vi "Setup SMU Channels.vi"(0 "TSM context":T1) -> (15 "error out":errorcluster)   [LabVIEW 2019]
uses:
  <vilib>/NI_TestStand_SemiconductorModule/NI_TestStand_Semiconductor_Module.lvlibp/PinMap/General/SemiconductorModuleContext.ctl
  <instrlib>/niDCPower/nidcpower.llb/niDCPower Sense.ctl
  <instrlib>/niDCPower/nidcpower.llb/niDCPower Aperture Time Units.ctl
  <vilib>/Utility/High Resolution Polling Wait.vi
  Instrument Control/DCPower/SSC DCPower/Source/SSC DCPower Configure Output Connected.vi
  Instrument Control/DCPower/SSC DCPower/Source/SSC DCPower Configure Output Enabled.vi
  <vilib>/NI_TestStand_SemiconductorModule/NI_TestStand_Semiconductor_Module.lvlibp
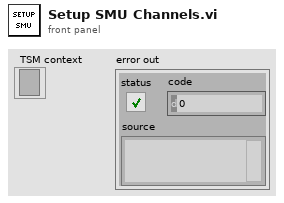
[diagram p1: front panel]
types:
  T1 = typedef "NI_TestStand_Semiconductor_Module.lvlibp/SemiconductorModuleContext.ctl" = refnum<k7>
  T2 = typedef "niDCPower Aperture Time Units.ctl" = i32
  T3 = typedef "niDCPower Sense.ctl" = i32
  T4 = typedef "TSM SSC DCPower.ctl" = cluster{"Pin Query Context":refnum<class "MultiplePinMultipleSessionQueryContext.lvclass">, "SSC":T5[], "Site Numbers":i32[], "Pins":T6[], "Pins Expanded":T8[]}
  T5 = typedef "SSC DCPower.ctl" = cluster{"Session":refnum<k15>, "Chan":string, "Channel List":string}
  T6 = typedef "TSM Pin Information.ctl" = cluster{"Pin":tag, "Type":T7, "Count":i32}
  T7 = typedef "TSM Pin Type Identifier.ctl" = enum8{"DUT Pin", "System Pin", "Pin Group", "Not Determined"}
  T8 = typedef "TSM Expanded Pin Information.ctl" = cluster{"Pin":tag, "Type":T7, "Index":i32}
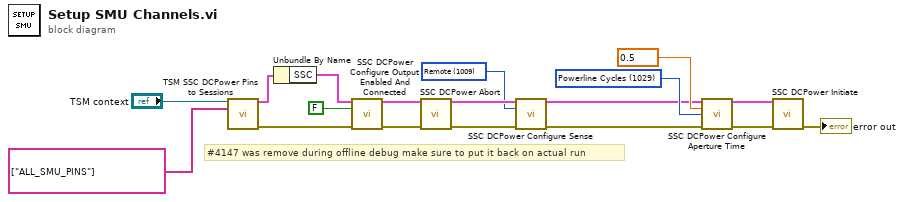
[diagram p0: block diagram]
diagram:
  w4 = T2 1029 items=["Seconds"=1028, "Powerline Cycles"=1029] ("Aperture Time Units")
  w8 = T3 1009 items=["Local"=1008, "Remote"=1009] ("Sense")
  # "#4147 was remove during offline debug make sure to put it back on actual run"
  n1 = call "TSM SSC DCPower Pins to Sessions.vi"("TSM context"="TSM context", "Pins"=tag[] ["ALL_SMU_PINS"]) -> ("DCPower TSM Out"=w15:T4, "error out"=w16:errorcluster)  [unwired: 12 in]
  n2 = Unbundle By Name(w15) -> ("SSC"=w14:T5[])
  n3 = call "SSC DCPower Configure Output Enabled And Connected.vi"("DCPower SSC in"=w14, "Output Enabled And Connected"=FALSE, "error in"=w16) -> ("DCPower SSC out"=w11:T5[], "error out"=w12:errorcluster)  [unwired: 11 in]
  n4 = call "SSC DCPower Abort.vi"("DCPower SSC in"=w11, "error in"=w12) -> ("DCPower SSC out"=w9:T5[], "error out"=w10:errorcluster)  [unwired: 12 in]
  n5 = call "SSC DCPower Configure Sense.vi"("DCPower SSC in"=w9, "Sense"=w8, "error in"=w10) -> ("DCPower SSC out"=w1:T5[], "error out"=w7:errorcluster)  [unwired: 11 in]
  n6 = call "SSC DCPower Configure Aperture Time.vi"("DCPower SSC in"=w1, "Aperture Time"=0.5, "Aperture Time Units"=w4, "error in"=w7) -> ("DCPower SSC out"=w2:T5[], "error out"=w5:errorcluster)  [unwired: 10 in]
  n7 = call "SSC DCPower Initiate.vi"("DCPower SSC in"=w2, "error in"=w5) -> ("error out"=→"error out":errorcluster)  [unwired: 12 in, 1 out]
